vi "Event Handler.vi"(8 "error in (no error)":errorcluster, 10 "Stop Event Handler":refnum<user-event>, 11 "path-with-auto-complete in":refnum<class "path-with-auto-complete.lvclass">) -> (0 "error out":errorcluster)   [LabVIEW 2020, in "path-with-auto-complete.lvclass"]
doc: "The <b>Event Handler VI</b> is a dynamic dispatch VI that should be overwritten if events are needed to create the enhanced QControl. \n\nBy inheriting from the main Control.lvclass the overwritten <b>Event Handler VI</b> will be launched asynchronously in the initialization of the QControl.\n<b> </b> <b> </b>\n©2016 Q Software Innovations, LLC (QSI)\nwritten by Quentin Alldredge\nproduced in LabVIEW 2015\n\nsupport@qsoftwareinnovations.com\nwww.qsoftwareinnovations.com\n\nAll rights reserved.\n\nRedistribution and use in source and binary forms, with or without modification, are permitted provided that the following conditions are met:\n\n * Redistributions of source code must retain the above copyright notice, this list of conditions and the following disclaimer.\n * Redistributions in binary form must reproduce the above copyright notice, this list of conditions and the following disclaimer in the documentation and/or other materials provided with the distribution.\n * Neither the name of Q Software Innovations, LLC. nor the names of its contributors may be used to endorse or promote products derived from this software without specific prior written permission.\n\nTHIS SOFTWARE IS PROVIDED BY THE COPYRIGHT HOLDERS AND CONTRIBUTORS \"AS IS\" AND ANY EXPRESS OR IMPLIED WARRANTIES, INCLUDING, BUT NOT LIMITED TO, THE IMPLIED WARRANTIES OF MERCHANTABILITY AND FITNESS FOR A PARTICULAR PURPOSE ARE DISCLAIMED. IN NO EVENT SHALL THE COPYRIGHT OWNER OR CONTRIBUTORS BE LIABLE FOR ANY DIRECT, INDIRECT, INCIDENTAL, SPECIAL, EXEMPLARY, OR CONSEQUENTIAL DAMAGES (INCLUDING, BUT NOT LIMITED TO, PROCUREMENT OF SUBSTITUTE GOODS OR SERVICES; LOSS OF USE, DATA, OR PROFITS; OR BUSINESS INTERRUPTION) HOWEVER CAUSED AND ON ANY THEORY OF LIABILITY, WHETHER IN CONTRACT, STRICT LIABILITY, OR TORT (INCLUDING NEGLIGENCE OR OTHERWISE) ARISING IN ANY WAY OUT OF THE USE OF THIS SOFTWARE, EVEN IF ADVISED OF THE POSSIBILITY OF SUCH DAMAGE."
uses:
  path-with-auto-complete.lvclass
  path-with-auto-complete.lvclass/path-with-auto-complete.ctl
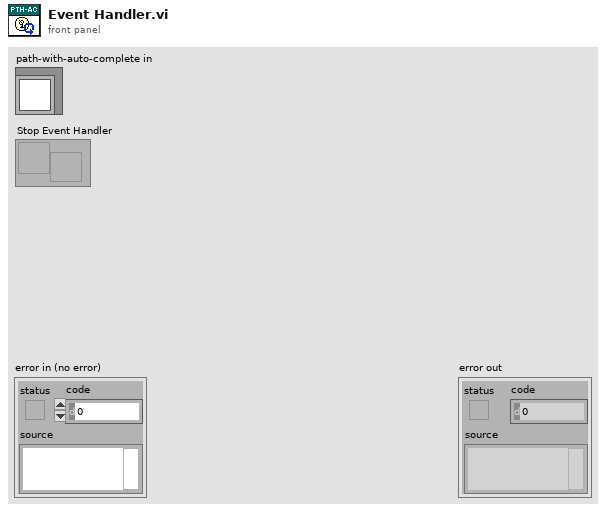
[diagram p1: front panel]
types:
  T1 = typedef "path-with-auto-complete.lvclass/State Data.ctl" = cluster{"Data":bool, "debug":bool, "mouse-down":bool, "has-focus":bool}
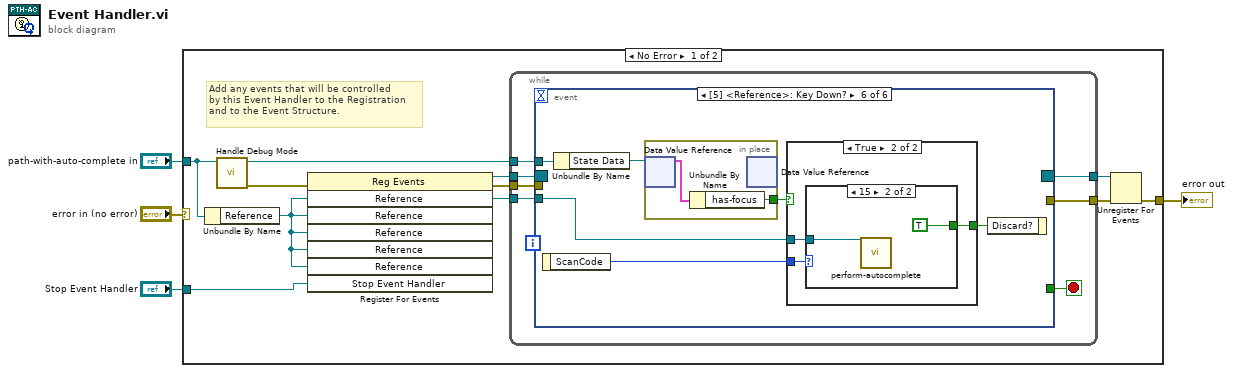
[diagram p0: block diagram]
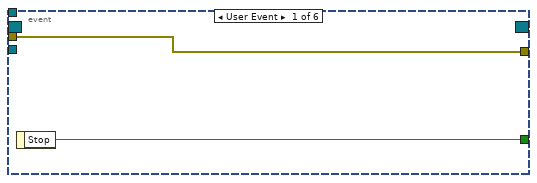
[diagram p2: hidden frame]
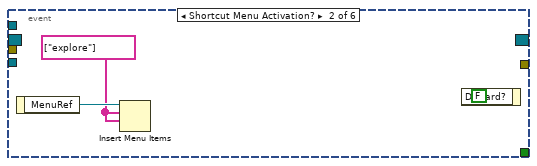
[diagram p3: hidden frame]
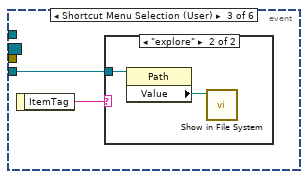
[diagram p4: hidden frame]
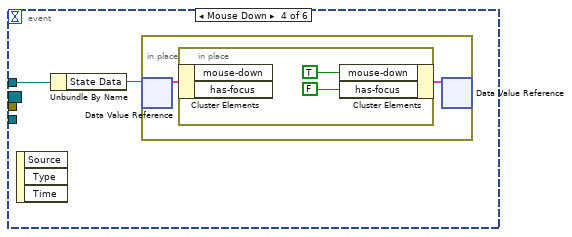
[diagram p6: hidden frame]
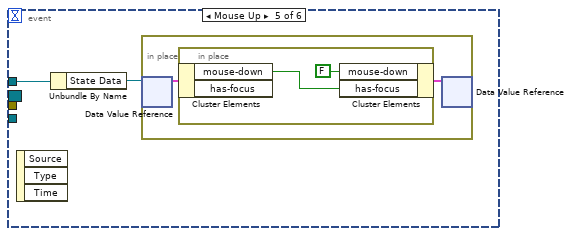
[diagram p7: hidden frame]
diagram:
  n1 = case shown="No Error" "error in (no error)" {
    selector: "error in (no error)" -> [_ w56]
    tunnel: [w11 w56] -> w3
    tunnel: "path-with-auto-complete in" -> [w7 _]
    tunnel: "Stop Event Handler" -> [w9 _]
    frame No Error {
      # "Add any events that will be controlled\nby this Event Handler to the Registration\nand to the Event Structure."
      n2 = Unbundle By Name(w7) -> ("Reference"=w8:refnum<vi>)
      n3 = call "Handle Debug Mode.vi"("path-with-auto-complete in"=w7) -> ("error out"=w6:errorcluster, "path-with-auto-complete out"=w5:refnum<class "path-with-auto-complete.lvclass">)  [unwired: 9 in]
      n4 = register-events(error in=w6, w8, w8, w8, w8, w8, w9) -> (reference out=w14:refnum<event-registration>, error out=w13:errorcluster)  [unwired: 1 in]
      n5 = while {
        tunnel: w14 -> [w21]
        tunnel: w13 -> [w19]
        tunnel: [w18] -> w12
        tunnel: [w16] -> w10
        tunnel: w8 -> [w15]
        tunnel: w5 -> [w20]
        stop <- w17 stop-if-true
        n6 = event shown="[5] <Reference>: Key Down?" {
          selector: w21 -> [_ _ _ _ _ _]
          dyn-events: [_ _ _ _ _ _] -> w16
          timeout: _ -> [_ _ _ _ _ _]
          tunnel: w20 -> [_ _ _ w32 w38 w48]
          tunnel: w19 -> [w23 _ _ _ _ _]
          tunnel: [w23 _ _ _ _ _] -> w18
          tunnel: [w22 _ _ _ _ _] -> w17
          tunnel: w15 -> [_ _ w27 _ _ w44]
          event User Event {
            n7 = event-data() -> ("Stop"=w22:bool)  [unwired: 1 in]
          }
          event Shortcut Menu Activation? {
            w25 = string[] ["explore"] ("item names")
            n8 = event-data() -> ("MenuRef"=w26:refnum<k9>)  [unwired: 1 in]
            n9 = Insert Menu Items(7:w25, 8:w25, 9:w26) -> ()  [unwired: 3 in, 3 out]
            n10 = event-data("Discard?"=FALSE) -> ()  [unwired: 1 in, 1 out]
          }
          event Shortcut Menu Selection (User) {
            n11 = event-data() -> ("ItemTag"=w28:string)  [unwired: 1 in]
            n12 = case shown="\"explore\"" w28 {
              tunnel: w27 -> [_ w30]
              frame Default {
              }
              frame "explore" {
                n13 = property class="Path"(reference=w30) -> ("Value"=w29:path)  [unwired: 1 in, 2 out]
                n14 = call <vilib>:"Show in File System.vi"("file or directory path"=w29) -> ()  [unwired: 10 in, 1 out]
              }
            }
          }
          event Mouse Down {
            n15 = event-data() -> ()  [unwired: 1 in, 3 out]
            n16 = Unbundle By Name(w32) -> ("State Data"=w31:refnum<data-value>)
            n17 = in-place {
              n18 = in-place-dvr #1(w31) -> (w34:T1)  [unwired: 1 out]
              n19 = in-place {
                n20 = in-place-cluster #2(w34) -> ()  [unwired: 2 out]
                n21 = in-place-cluster #2("mouse-down"=TRUE ("key-down"), "has-focus"=FALSE ("key-down")) -> (w33:T1)
              }
              n22 = in-place-dvr #1(w33) -> ()  [unwired: 2 out]
            }
          }
          event Mouse Up {
            n23 = event-data() -> ()  [unwired: 1 in, 3 out]
            n24 = Unbundle By Name(w38) -> ("State Data"=w37:refnum<data-value>)
            n25 = in-place {
              n26 = in-place-dvr #3(w37) -> (w40:T1)  [unwired: 1 out]
              n27 = in-place {
                n28 = in-place-cluster #4(w40) -> ("mouse-down"=w42:bool)  [unwired: 1 out]
                n29 = in-place-cluster #4("mouse-down"=FALSE, "has-focus"=w42) -> (w39:T1)
              }
              n30 = in-place-dvr #3(w39) -> ()  [unwired: 2 out]
            }
          }
          event Key Down? {
            n31 = event-data() -> ("ScanCode"=w46:i16)  [unwired: 1 in]
            n32 = Unbundle By Name(w48) -> ("State Data"=w47:refnum<data-value>)
            n33 = in-place {
              in-place-border: [w55] -> w45
              n34 = in-place-dvr #5(w47) -> (w54:T1)  [unwired: 1 out]
              n35 = Unbundle By Name(w54) -> ("has-focus"=w55:bool)
              n36 = in-place-dvr #5() -> ()  [unwired: 1 in, 2 out]
            }
            n37 = case shown="True" w45 {
              tunnel: w46 -> [_ w51]
              tunnel: w44 -> [_ w50]
              tunnel: [_ w49] -> w43
              frame False {
              }
              frame True {
                n38 = case shown="15" w51 {
                  tunnel: w50 -> [_ w53]
                  tunnel: [_ TRUE ("Discard?")] -> w49
                  frame Default {
                  }
                  frame 15 {
                    n39 = call "perform-autocomplete.vi"("Path in"=w53) -> ()  [unwired: 11 in]
                  }
                }
              }
            }
            n40 = event-data("Discard?"=w43) -> ()  [unwired: 1 in, 1 out]
          }
        }
      }
      n41 = Unregister For Events(event registration refnum=w10, error in=w12) -> (error out=w11:errorcluster)
    }
    frame Error {
    }
  }
  "error out" <- w3
